vi "SaveText.vi"(7 "action":string="Save", 8 "error in":errorcluster, 9 "GAIN":sgl=100.0, 10 "data in":sgl, 11 "file path (use dialog)":path) -> (0 "error out":errorcluster)   [LabVIEW 2018]
uses:
  <vilib>/Utility/file.llb/Write Delimited Spreadsheet (DBL).vi
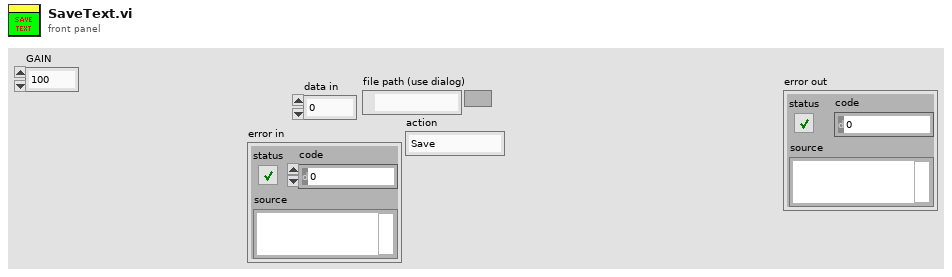
[diagram p1: front panel]
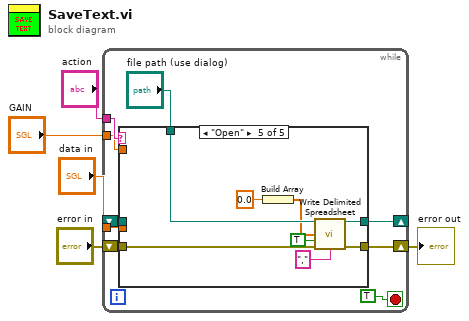
[diagram p0: block diagram]
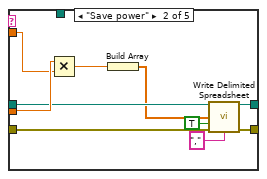
[diagram p3: hidden frame]
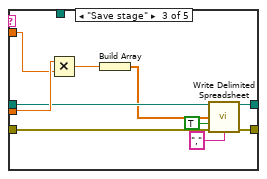
[diagram p4: hidden frame]
diagram:
  n1 = while {
    tunnel: "action" -> [w13]
    tunnel: "data in" -> [w12]
    shift-right: [w10] -> w2
    shift-left: "error in" -> [w11]
    tunnel: "GAIN" -> [w9]
    shift-right: [w8] -> _
    shift-left: _ -> [w6]
    stop <- TRUE stop-if-true
    n2 = case shown="\"Open\"" w13 {
      tunnel: w12 -> [_ w24 w34 _ _]
      tunnel: w11 -> [w16 w26 w36 w37 w44]
      tunnel: [w16 w25 w35 w37 w45] -> w10
      tunnel: w9 -> [_ w23 w33 _ _]
      tunnel: [w15 w19 w31 _ w43] -> w8
      tunnel: "file path (use dialog)" -> [_ _ _ _ w42]
      tunnel: w6 -> [w15 w22 w32 _ _]
      frame "False", Default {
      }
      frame "Save power" {
        n3 = Multiply(x=w24, y=w23) -> (x*y=w21:sgl)
        n4 = Build Array(w21) -> (w20:sgl[])
        n5 = call-poly <vilib>:"Write Delimited Spreadsheet.vi"("file path (dialog if empty)"=w22, "1D data"=w20, "append to file? (new file:F)"=TRUE, "error in (no error)"=w26, "delimiter (\\t)"="," ("delimiter (\\t)")) -> ("new file path (Not A Path if cancelled)"=w19:path, "error out"=w25:errorcluster)  [unwired: 9 in]
      }
      frame "Save stage" {
        n6 = Multiply(x=w34, y=w33) -> (x*y=w30:sgl)
        n7 = Build Array(w30) -> (w29:sgl[])
        n8 = call-poly <vilib>:"Write Delimited Spreadsheet.vi"("file path (dialog if empty)"=w32, "1D data"=w29, "append to file? (new file:F)"=TRUE, "error in (no error)"=w36, "delimiter (\\t)"="," ("delimiter (\\t)")) -> ("new file path (Not A Path if cancelled)"=w31:path, "error out"=w35:errorcluster)  [unwired: 9 in]
      }
      frame "Close" {
      }
      frame "Open" {
        n9 = Build Array(0.0 ("element")) -> (w39:dbl[])
        n10 = call-poly <vilib>:"Write Delimited Spreadsheet.vi"("file path (dialog if empty)"=w42, "1D data"=w39, "append to file? (new file:F)"=TRUE, "error in (no error)"=w44, "delimiter (\\t)"="," ("delimiter (\\t)")) -> ("new file path (Not A Path if cancelled)"=w43:path, "error out"=w45:errorcluster)  [unwired: 9 in]
      }
    }
  }
  "error out" <- w2
